vi "pp2_DAQclear.vi"(8 "error in (no error)":errorcluster, 11 "Daq config in":T1={"Sound AO"="Dev2/ao0", "Shock intesity AO"="Dev1/ao1", "Code_LED DO"="Dev1/port1:2", "Switch DI"="Dev1/port0/line0:1", "Webcam"="cam0", "Sound AO task"="", "Sound card task"=0, "Shock intensity AO task"="", "Code_LED DO task"="", "Switch DI task"="", "AO <=> Sound card"=FALSE, "Sound card"=0, "sample rate"=8000.0, "Variable shock"=FALSE, "Webcam on"=FALSE, "Tone gate PFI"="/Dev1/PFI1", "Waveform memo"={"t0"=timestamp(0 s since 1904-01-01), "dt"=1.0, "Y"=[]}, "First time"=FALSE} {"sample rate" min=8000.0; "Sound card task" format="%.0x"}) -> (0 "error out":errorcluster, 3 "Daq config out":T1={"Sound AO"="Dev2/ao0", "Shock intesity AO"="Dev1/ao1", "Code_LED DO"="Dev1/port1:2", "Switch DI"="Dev1/port0/line0:1", "Webcam"="cam0", "Sound AO task"="", "Sound card task"=0, "Shock intensity AO task"="", "Code_LED DO task"="", "Switch DI task"="", "AO <=> Sound card"=FALSE, "Sound card"=0, "sample rate"=8000.0, "Variable shock"=FALSE, "Webcam on"=FALSE, "Tone gate PFI"="/Dev1/PFI1", "Waveform memo"={"t0"=timestamp(0 s since 1904-01-01), "dt"=1.0, "Y"=[]}, "First time"=FALSE} {"sample rate" min=8000.0; "Sound card task" format="%.0x"})   [LabVIEW 2013]
uses:
  pp2_CTL_DaqConfig.ctl
  <vilib>/userdefined/High Color/IMAQdx.ctl
  <vilib>/sound2/lvsound2.llb/Sound Output Task ID.ctl
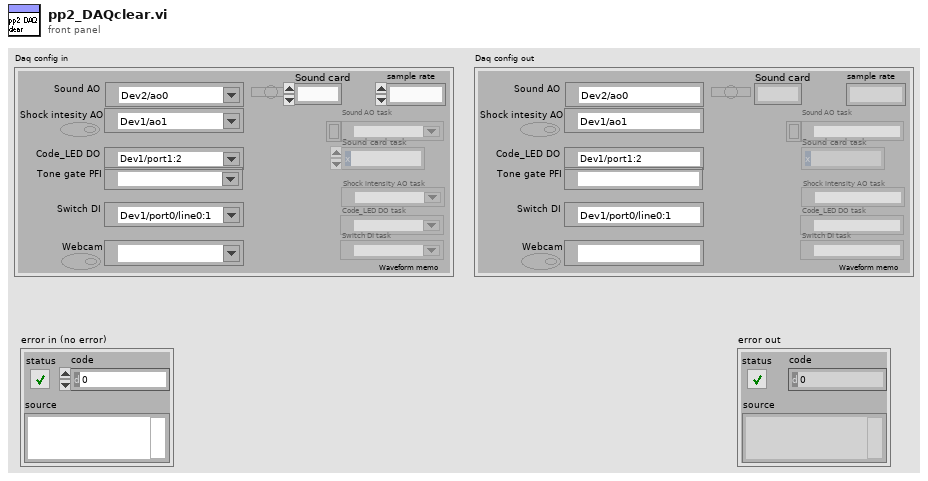
[diagram p1: front panel]
types:
  T1 = typedef "pp2_CTL_DaqConfig.ctl" = cluster{"Sound AO":tag, "Shock intesity AO":tag, "Code_LED DO":tag, "Switch DI":tag, "Webcam":T2, "Sound AO task":refnum<k21>, "Sound card task":T3, "Shock intensity AO task":refnum<k21>, "Code_LED DO task":refnum<k21>, "Switch DI task":refnum<k21>, "AO <=> Sound card":bool, "Sound card":u32, "sample rate":dbl, "Variable shock":bool, "Webcam on":bool, "Tone gate PFI":tag, "Waveform memo":waveform(dbl), "First time":bool}
  T2 = typedef "IMAQdx.ctl" = refnum<k21>
  T3 = typedef "Sound Output Task ID.ctl" = u32
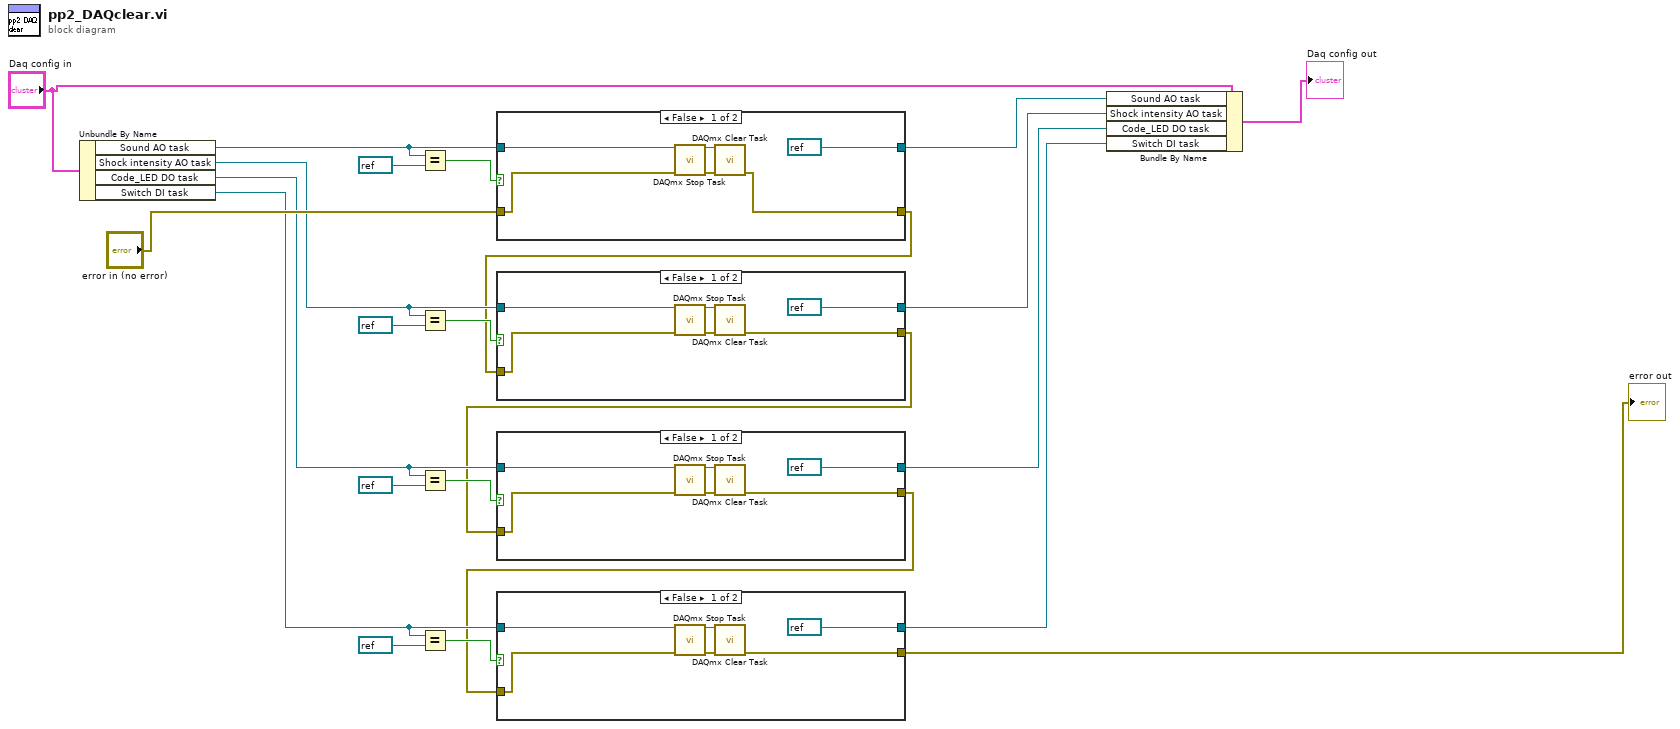
[diagram p0: block diagram]
diagram:
  n1 = Unbundle By Name("Daq config in") -> ("Sound AO task"=w12:refnum<k21>, "Shock intensity AO task"=w7:refnum<k21>, "Code_LED DO task"=w6:refnum<k21>, "Switch DI task"=w5:refnum<k21>)
  n2 = Equal?(x=w12, y=refnum<k21> refnum) -> (x = y?=w22:bool)
  n3 = Equal?(x=w7, y=refnum<k21> refnum) -> (x = y?=w17:bool)
  n4 = Equal?(x=w6, y=refnum<k21> refnum) -> (x = y?=w15:bool)
  n5 = Equal?(x=w5, y=refnum<k21> refnum) -> (x = y?=w13:bool)
  n6 = case shown="False" w22 {
    tunnel: w12 -> [w27 w31]
    tunnel: [refnum<k21> refnum ("NULL") w31] -> w21
    tunnel: "error in (no error)" -> [w26 w30]
    tunnel: [w24 w30] -> w4
    frame False {
      n7 = call <vilib>:"DAQmx Stop Task.vi"("task/channels in"=w27, "error in"=w26) -> ("task out"=w29:refnum<k21>, "error out"=w28:errorcluster)  [unwired: 12 in]
      n8 = call <vilib>:"DAQmx Clear Task.vi"("task in"=w29, "error in"=w28) -> ("error out"=w24:errorcluster)  [unwired: 13 in]
    }
    frame True {
    }
  }
  n9 = case shown="False" w17 {
    tunnel: w7 -> [w35 w39]
    tunnel: [refnum<k21> refnum ("NULL") w39] -> w10
    tunnel: w4 -> [w34 w38]
    tunnel: [w32 w38] -> w3
    frame False {
      n10 = call <vilib>:"DAQmx Stop Task.vi"("task/channels in"=w35, "error in"=w34) -> ("task out"=w37:refnum<k21>, "error out"=w36:errorcluster)  [unwired: 12 in]
      n11 = call <vilib>:"DAQmx Clear Task.vi"("task in"=w37, "error in"=w36) -> ("error out"=w32:errorcluster)  [unwired: 13 in]
    }
    frame True {
    }
  }
  n12 = case shown="False" w15 {
    tunnel: w6 -> [w43 w47]
    tunnel: [refnum<k21> refnum ("NULL") w47] -> w9
    tunnel: w3 -> [w42 w46]
    tunnel: [w40 w46] -> w2
    frame False {
      n13 = call <vilib>:"DAQmx Stop Task.vi"("task/channels in"=w43, "error in"=w42) -> ("task out"=w45:refnum<k21>, "error out"=w44:errorcluster)  [unwired: 12 in]
      n14 = call <vilib>:"DAQmx Clear Task.vi"("task in"=w45, "error in"=w44) -> ("error out"=w40:errorcluster)  [unwired: 13 in]
    }
    frame True {
    }
  }
  n15 = case shown="False" w13 {
    tunnel: w5 -> [w51 w55]
    tunnel: [refnum<k21> refnum ("NULL") w55] -> w8
    tunnel: w2 -> [w50 w54]
    tunnel: [w48 w54] -> w1
    frame False {
      n16 = call <vilib>:"DAQmx Stop Task.vi"("task/channels in"=w51, "error in"=w50) -> ("task out"=w53:refnum<k21>, "error out"=w52:errorcluster)  [unwired: 12 in]
      n17 = call <vilib>:"DAQmx Clear Task.vi"("task in"=w53, "error in"=w52) -> ("error out"=w48:errorcluster)  [unwired: 13 in]
    }
    frame True {
    }
  }
  "error out" <- w1
  n18 = Bundle By Name(cluster="Daq config in", "Sound AO task"=w21, "Shock intensity AO task"=w10, "Code_LED DO task"=w9, "Switch DI task"=w8) -> (→"Daq config out":T1)
